vi "HIOKI PW3390 Meas Integ Start.vi"(0 "VISA Resource":refnum<visa-resource-name>, 11 "error in (no error)":errorcluster, 12 "OPC query (T: ON)":bool=TRUE, 13 "Error Out (F: Off)":bool) -> (4 "VISA Resource out":refnum<visa-resource-name>, 15 "error out":errorcluster)   [LabVIEW 2009]
doc: "Starts Integration (time control)."
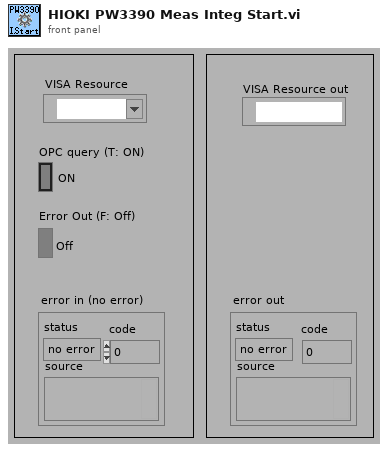
[diagram p1: front panel]
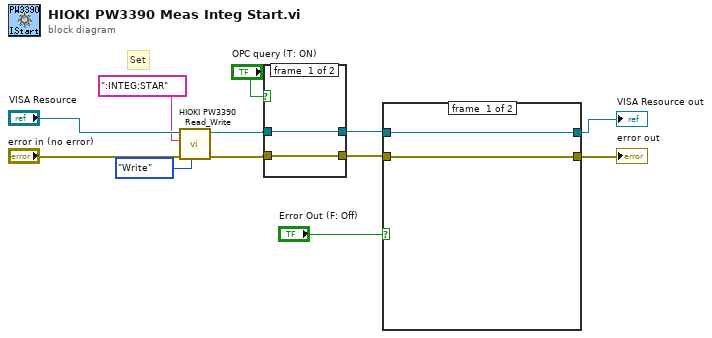
[diagram p0: block diagram]
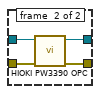
[diagram p2: hidden frame]
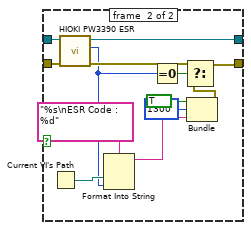
[diagram p3: hidden frame]
diagram:
  # "Set"
  n1 = call <instrlib>:"HIOKI PW3390 Read_Write.vi"("Read/Write"=enum16{"Read", "Write"}."Write", "error in (no error)"="error in (no error)", "data in"=":INTEG:STAR", "VISA Resource"="VISA Resource") -> ("error out"=w3:errorcluster, "VISA Resource out"=w4:refnum<visa-resource-name>)  [unwired: 5 in, 1 out]
  n2 = case shown="TRUE" "OPC query (T: ON)" {
    tunnel: [w14 w18] -> w2
    tunnel: [w13 w17] -> w1
    tunnel: w4 -> [w14 w16]
    tunnel: w3 -> [w13 w15]
    frame #0 {
    }
    frame #1 {
      n3 = call <instrlib>:"HIOKI PW3390 OPC.vi"("error in (no error)"=w15, "VISA Resource"=w16) -> ("error out"=w17:errorcluster, "VISA Resource out"=w18:refnum<visa-resource-name>)  [unwired: 7 in, 1 out]
    }
  }
  n4 = case shown="TRUE" "Error Out (F: Off)" {
    tunnel: w2 -> [w20 w33]
    tunnel: w1 -> [w19 w32]
    tunnel: [w19 w22] -> w9
    tunnel: [w20 w31] -> w6
    frame #0 {
    }
    frame #1 {
      n5 = Current VI's Path() -> (path=w29:path)
      n6 = call <instrlib>:"HIOKI PW3390 ESR.vi"("error in (no error)"=w32, "VISA Resource"=w33) -> ("error out"=w23:errorcluster, "Output Value"=w21:u8, "VISA Resource out"=w31:refnum<visa-resource-name>)  [unwired: 6 in, 1 out]
      n7 = Format Into String(format string="%s\nESR Code : %d", w29, w21) -> (resulting string=w25:string)  [unwired: 2 in, 1 out]
      n8 = Equal To 0?(x=w21) -> (x = 0?=w30:bool)
      n9 = Bundle("status"=TRUE, "code"=1300, w25) -> (w24:cluster{"status":bool, "code":i32, string})  [unwired: 1 in]
      n10 = Select(t=w23, s=w30, f=w24) -> (s? t:f=w22:errorcluster)
    }
  }
  "error out" <- w9
  "VISA Resource out" <- w6
